vi "GDSString_GetModifiers.vi"(8 "error in (no error)":errorcluster, 10 "DefaultAccesssScopr(Public)":T1, 11 "Words":string[](array[string])) -> (0 "error out":errorcluster, 2 "Array out":T2[](array[typedef]), 3 "AccessScope":T1)   [LabVIEW 2012]
uses:
  <resource>/Framework/Providers/Open_GDS/ClassProviders/Common/String/GDSString_AccessScopeModifierType.ctl
  <resource>/Framework/Providers/Open_GDS/ClassProviders/Common/String/GDSString_ModifierType.ctl
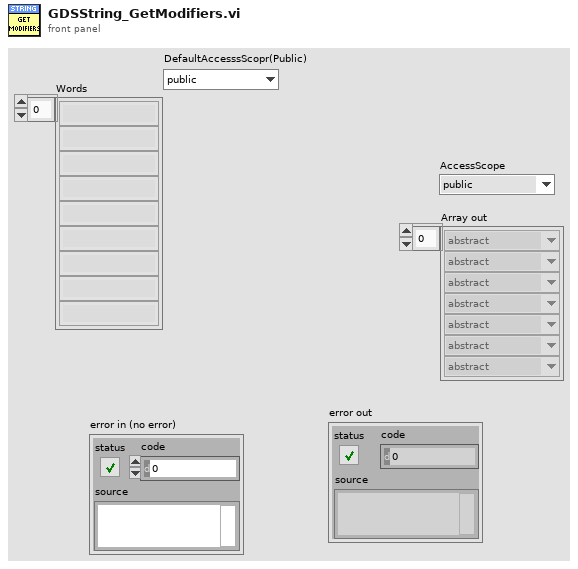
[diagram p1: front panel]
types:
  T1 = typedef "GDSString_AccessScopeModifierType.ctl" = enum16{"public", "private", "protected", "internal"}
  T2 = typedef "GDSString_ModifierType.ctl" = enum16{"abstract", "static", "final", "synchronized", "strictfp", "async", "const", "event", "extern", "new", "native ", "override", "partial", "readonly", "sealed", "unsafe", "virtual", "volatile"}
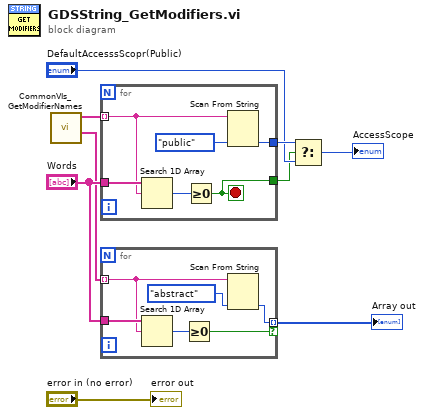
[diagram p0: block diagram]
diagram:
  n1 = call <resource>:"CommonVIs_GetModifierNames.vi"() -> ("ExatrModifiers"=w1:string[], "AccessScopeModifiers"=w2:string[])  [unwired: 9 in, 1 out]
  n2 = for {
    tunnel: "Words" -> [w14]
    tunnel: [w12] -> w9
    tunnel: [w11] -> w6
    tunnel: w2 -> [w10] mode=indexing
    stop <- w11 stop-if-true
    n3 = Search 1D Array(1D array=w14, element=w10) -> (index of element=w15:i32)  [unwired: 1 in]
    n4 = Greater Or Equal To 0?(x=w15) -> (x >= 0?=w11:bool)
    n5 = Scan From String(input string=w10, default 1=GDSString_AccessScopeModifierType."public" ("AccessScope")) -> (output 1=w12:T1)  [unwired: 3 in, 3 out]
  }
  n6 = for {
    tunnel: "Words" -> [w20]
    tunnel: w1 -> [w16] mode=indexing
    tunnel: [w19] -> w5 mode=indexing if=w18
    n7 = Search 1D Array(1D array=w20, element=w16) -> (index of element=w21:i32)  [unwired: 1 in]
    n8 = Greater Or Equal To 0?(x=w21) -> (x >= 0?=w18:bool)
    n9 = Scan From String(input string=w16, default 1=GDSString_ModifierType."abstract" ("Modifiers")) -> (output 1=w19:T2)  [unwired: 3 in, 3 out]
  }
  "Array out" <- w5
  n10 = Select(t=w9, s=w6, f="DefaultAccesssScopr(Public)") -> (s? t:f=→"AccessScope":T1)
  "error out" <- "error in (no error)"
